vi "Act Inventario.vi"(8 "error in (no error)":errorcluster, 9 "Producto":string, 10 "Inventario":dbl, 11 "Coca Actor in":refnum<class "Coca Actor.lvclass">) -> (0 "error out":errorcluster, 3 "Coca Actor out":refnum<class "Coca Actor.lvclass">)   [LabVIEW 2020, in "Coca Actor.lvlib" / "Coca Actor.lvclass"]
uses:
  Coca Actor.lvclass
  <vilib>/Utility/config.llb/Write Key (Double).vi
  <vilib>/Utility/config.llb/NI_LVConfig.lvlib
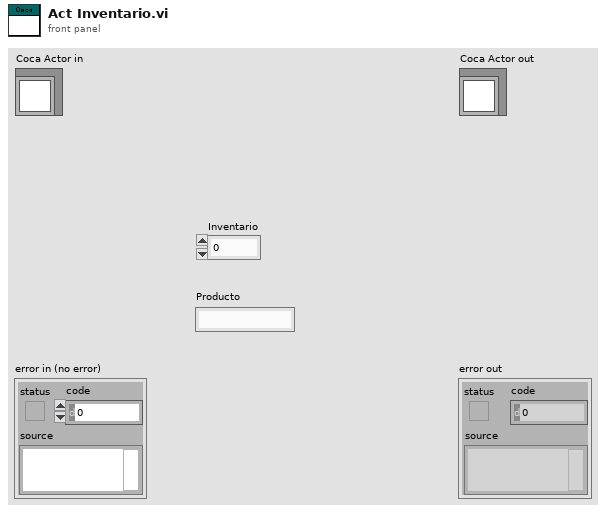
[diagram p1: front panel]
types:
  T1 = typedef "NI_LVConfig.lvlib/Config Data RefNum.ctl" = refnum<k1>
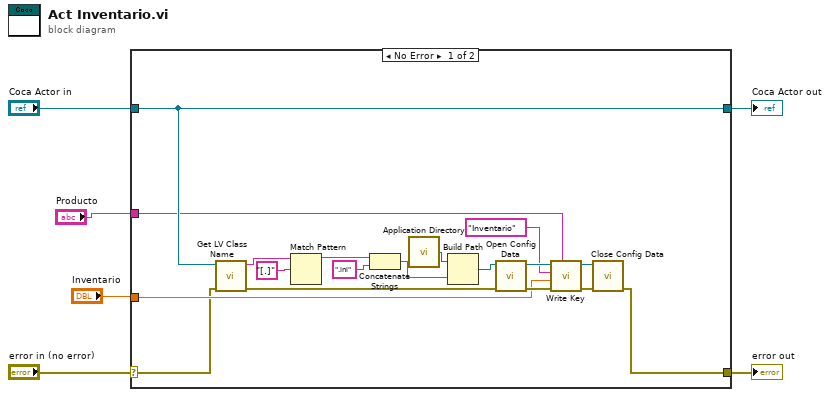
[diagram p0: block diagram]
diagram:
  n1 = case shown="No Error" "error in (no error)" {
    selector: "error in (no error)" -> [w8 w26]
    tunnel: [w7 w26] -> w5
    tunnel: [w11 w25] -> w3
    tunnel: "Coca Actor in" -> [w11 w25]
    tunnel: "Producto" -> [w10 _]
    tunnel: "Inventario" -> [w9 _]
    frame No Error {
      n2 = call <vilib>:"Get LV Class Name.vi"("error in (no error)"=w8, "object"=w11) -> ("error out"=w12:errorcluster, "class name"=w15:string)  [unwired: 8 in]
      n3 = Match Pattern(string=w15, regular expression="[.]") -> (before substring=w18:string)  [unwired: 1 in, 3 out]
      n4 = Concatenate Strings(w18, ".ini" ("string")) -> (w24:string)
      n5 = call <vilib>:"Application Directory.vi"() -> ("Application Directory"=w22:path)
      n6 = Build Path(base path=w22, name or relative path=w24) -> (appended path=w21:path)
      n7 = call <vilib>:"Open Config Data.vi"("error in (no error)"=w12, "configuration file path"=w21) -> ("error out"=w16:errorcluster, "refnum"=w17:T1)  [unwired: 7 in, 1 out]
      n8 = call-poly <vilib>:"Write Key.vi"("section"=w10, "error in (no error)"=w16, "value"=w9, "key"="Inventario", "refnum"=w17) -> ("error out"=w19:errorcluster, "refnum out"=w20:T1)  [unwired: 4 in, 1 out]
      n9 = call <vilib>:"Close Config Data.vi"("error in (no error)"=w19, "refnum"=w20) -> ("error out"=w7:errorcluster)  [unwired: 8 in, 1 out]
    }
    frame Error {
    }
  }
  "error out" <- w5
  "Coca Actor out" <- w3
